vi "Create Iterator.vi"(8 "error in (no error)":errorcluster caption="错误输入（无错误）", 11 "具体聚集 输入":refnum<class "具体聚集.lvclass"> caption="DNL_LabVIEW Object in") -> (0 "error out":errorcluster caption="错误输出", 2 "迭代器.lvlib:迭代器(抽象类).lvclass":refnum<class "迭代器(抽象类).lvclass">, 3 "具体聚集 输出":refnum<class "具体聚集.lvclass"> caption="DNL_LabVIEW Object out")   [LabVIEW 2011, in "迭代器.lvlib" / "具体聚集.lvclass"]
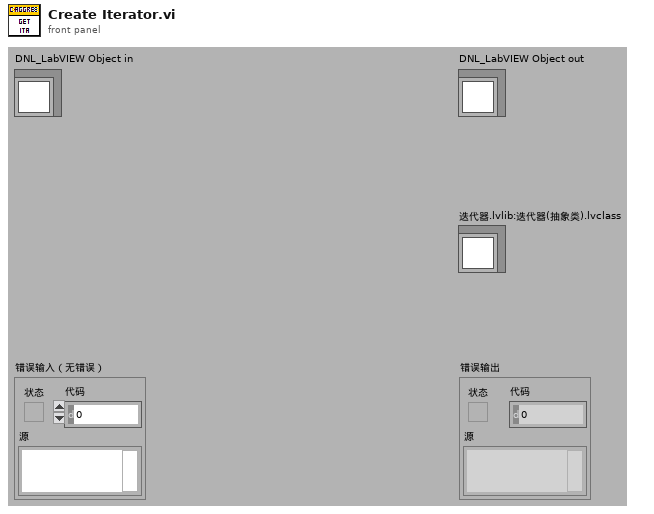
[diagram p1: front panel]
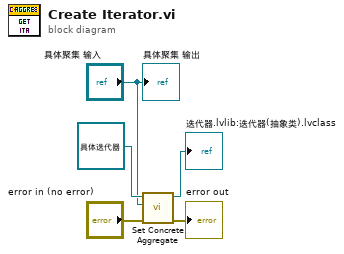
[diagram p0: block diagram]
diagram:
  n1 = call "Set Concrete Aggregate.vi"("error in (no error)"="error in (no error)", "迭代器.lvlib:具体聚集.lvclass"="具体聚集 输入", "具体迭代器 输入"=refnum<class "具体迭代器.lvclass"> refnum) -> ("error out"=→"error out":errorcluster, "具体迭代器 输出"=→"迭代器.lvlib:迭代器(抽象类).lvclass":refnum<class "具体迭代器.lvclass">)  [unwired: 7 in]
  "具体聚集 输出" <- "具体聚集 输入"
